vi "Voltage Ramp Text In.vi"(1 "command text in":string[](array[string])=["N/A", "Magent PS", "N/A", "Set Field", "Set Field to 2.0000E+0 @ 0.0000T /min, no wait , extra 0 sec wait", "N/A", "N/A", "", "1", "0", "N/A", "2.000000", "0.000000", "N/A", "N/A", "N/A", "N/A", "N/A", "N/A", "N/A", "N/A", "N/A", "N/A", "N/A", "N/A", "N/A", "N/A", "N/A", "N/A", "N/A", "N/A", "N/A", "N/A", "N/A"]) -> (0 "VoltageRamp":T1={"VISA Resource Name"="", "extra wait"=1, "start"=1e-12, "end"=0.002, "Sweep Time (H:M:S)"=1800.0, "Log Linear"=FALSE, "interval(sec)"=0.5, "Select instrument"=enum."Yokogawa GS200 Coarse"} {"interval(sec)" min=0.5 step=0.1; "Sweep Time (H:M:S)" format="%<%H:%M:%S>t"; "extra wait" min=0; "start" format="%#.7e"; "end" format="%#.7e"})   [LabVIEW 2021]
uses:
  VoltageRamp.ctl
  VoltageRamp Instrument.ctl
panel:
  # "Voltage Ramp"
  # "Select\nInstrument"
  # "Instrument \nAddress"
  # "Log"
  # "End Voltage (V)"
  # "Sweep Time (HH:MM:SS)"
  # "Start Voltage (V)"
  # "Linear"
  # "seconds"
  # "Minimum Time Interval Between Two Points"
  # "seconds"
  # "AND wait extra"
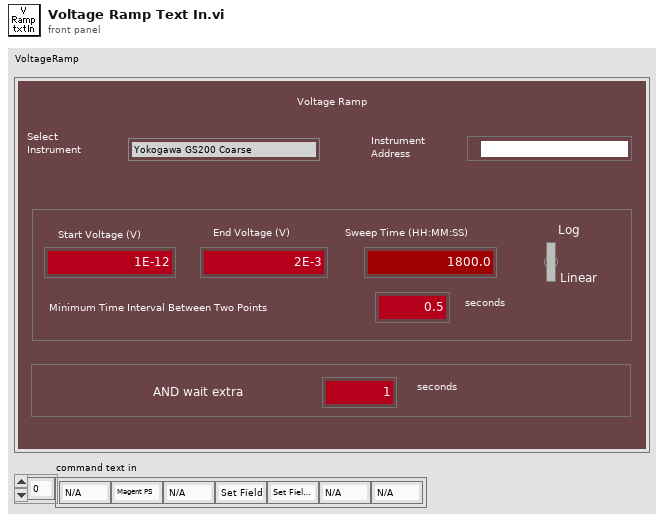
[diagram p1: front panel]
types:
  T1 = typedef "VoltageRamp.ctl" = cluster{"VISA Resource Name":refnum<visa-resource-name>, "extra wait":i32, "start":dbl, "end":dbl, "Sweep Time (H:M:S)":dbl, "Log Linear":bool, "interval(sec)":dbl, "Select instrument":T2}
  T2 = typedef "VoltageRamp Instrument.ctl" = enum16{"Yokogawa GS200 Coarse", "Keithley 24xx Coarse", "Keithley 230"}
  T3 = cluster{"command text in[0]":string, "command text in[1]":string, "command text in[2]":string, "command text in[3]":string, "command text in[4]":string, "command text in[5]":string, "command text in[6]":string, "command text in[7]":string, "command text in[8]":string, "command text in[9]":string, "command text in[10]":string, "command text in[11]":string, "command text in[12]":string, "command text in[13]":string, "command text in[14]":string, "command text in[15]":string, "command text in[16]":string, "command text in[17]":string, "command text in[18]":string, "command text in[19]":string, "command text in[20]":string, "command text in[21]":string}
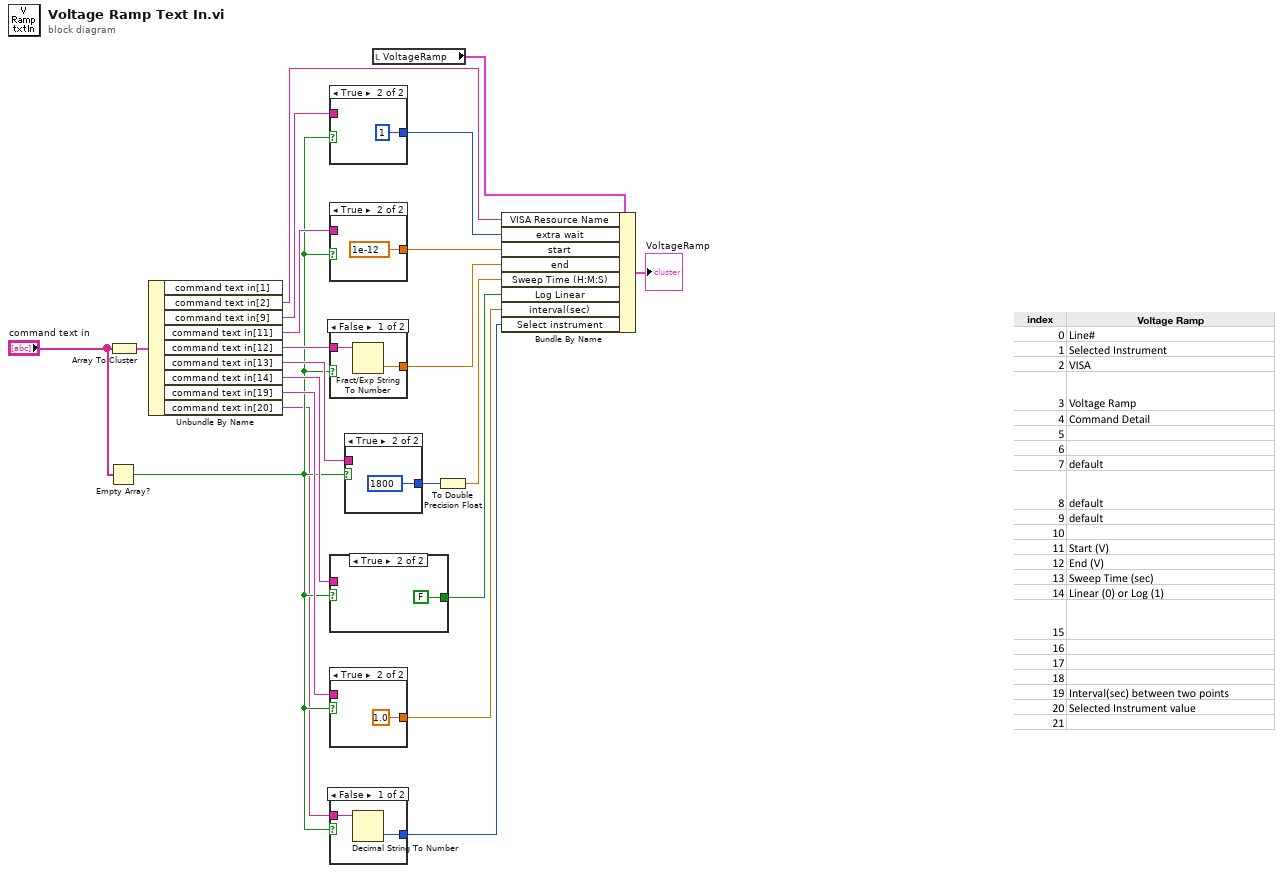
[diagram p0: block diagram]
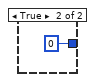
[diagram p2: hidden frame]
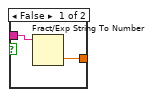
[diagram p3: hidden frame]
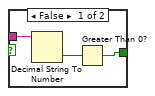
[diagram p4: hidden frame]
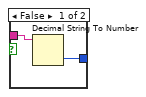
[diagram p5: hidden frame]
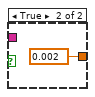
[diagram p6: hidden frame]
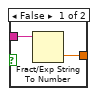
[diagram p7: hidden frame]
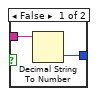
[diagram p8: hidden frame]
diagram:
  n1 = Empty Array?(array="command text in") -> (empty?=w3:bool)
  n2 = Array To Cluster(array="command text in") -> (cluster=w21:T3)
  n3 = Unbundle By Name(w21) -> ("command text in[2]"=w19:string, "command text in[9]"=w18:string, "command text in[11]"=w16:string, "command text in[12]"=w14:string, "command text in[13]"=w12:string, "command text in[14]"=w9:string, "command text in[19]"=w5:string, "command text in[20]"=w2:string)  [unwired: 1 out]
  n4 = case shown="True" w3 {
    tunnel: w18 -> [w23 _]
    tunnel: [w22 u16 1 ("Value (Signaling)")] -> w17
    frame False {
      n5 = Decimal String To Number(string=w23) -> (number=w22:i32)  [unwired: 2 in, 1 out]
    }
    frame True {
    }
  }
  n6 = case shown="True" w3 {
    tunnel: [w26 1e-12] -> w15
    tunnel: w16 -> [w25 _]
    frame False {
      n7 = Fract/Exp String To Number(string=w25) -> (number=w26:dbl)  [unwired: 3 in, 1 out]
    }
    frame True {
    }
  }
  n8 = case shown="False" w3 {
    tunnel: [w29 0.002] -> w13
    tunnel: w14 -> [w28 _]
    frame False {
      n9 = Fract/Exp String To Number(string=w28) -> (number=w29:dbl)  [unwired: 3 in, 1 out]
    }
    frame True {
    }
  }
  n10 = case shown="True" w3 {
    tunnel: w9 -> [w33 _]
    tunnel: [w32 FALSE] -> w8
    frame False {
      n11 = Decimal String To Number(string=w33) -> (number=w31:i32)  [unwired: 2 in, 1 out]
      n12 = Greater Than 0?(x=w31) -> (x > 0?=w32:bool)
    }
    frame True {
    }
  }
  n13 = case shown="True" w3 {
    tunnel: [w36 1.0] -> w4
    tunnel: w5 -> [w35 _]
    frame False {
      n14 = Fract/Exp String To Number(string=w35) -> (number=w36:dbl)  [unwired: 3 in, 1 out]
    }
    frame True {
    }
  }
  n15 = case shown="False" w3 {
    tunnel: w2 -> [w39 _]
    tunnel: [w38 0] -> w1
    frame False {
      n16 = Decimal String To Number(string=w39) -> (number=w38:i32)  [unwired: 2 in, 1 out]
    }
    frame True {
    }
  }
  n17 = case shown="True" w3 {
    tunnel: w12 -> [w42 _]
    tunnel: [w41 1800] -> w11
    frame False {
      n18 = Decimal String To Number(string=w42) -> (number=w41:i32)  [unwired: 2 in, 1 out]
    }
    frame True {
    }
  }
  n19 = local read "VoltageRamp"() -> (w7:T1)
  n20 = To Double Precision Float(number=w11) -> (double precision float=w10:dbl)
  n21 = Bundle By Name(cluster=w7, "VISA Resource Name"=w19, "extra wait"=w17, "start"=w15, "end"=w13, "Sweep Time (H:M:S)"=w10, "Log Linear"=w8, "interval(sec)"=w4, "Select instrument"=w1) -> (→"VoltageRamp":T1)
